vi "IsolateError.vi"(8 "Err Line":i32=71, 9 "Number of lines":i32=71, 10 "start":i32=1390, 11 "Console in":string=">>> \n>>> \nHUB: sync filesystems\nHUB: soft reboot\nTraceback (most recent call last):\n  File \"main.py\", line 81, in <module>\nKeyboardInterrupt: \nMicroPython v1.14-875-g1ed8d92bd on 2021-04-23; LEGO Technic Small Hub with STM32F413xx\nType \"help()\" for more information.\n>>> \nHUB: sync filesystems\nHUB: soft reboot\nTraceback (most recent call last):\n  File \"main.py\", line 81, in <module>\nKeyboardInterrupt: \nMicroPython v1.14-875-g1ed8d92bd on 2021-04-23; LEGO Technic Small Hub with STM32F413xx\nType \"help()\" for more information.\n>>> \n>>> \n>>> \n>>> \n>>> >>> \nHUB: sync filesystems\nHUB: soft reboot\nTraceback (most recent call last):\n  File \"main.py\", line 71, in <module>\n  File \"Backpack_Code.py\", line 81, in ask\n  File \"Backpack_Code.py\", line 56, in upload\n  File \"Backpack_Code.py\", line 25, in read\nKeyboardInterrupt: \nMicroPython v1.14-875-g1ed8d92bd on 2021-04-23; LEGO Technic Small Hub with STM32F413xx\nType \"help()\" for more information.\n>>> \n>>> \n>>> hub.\n__class__       __name__        __version__     BACK\nBOTTOM          BT_VCP          FRONT           LEFT\nRIGHT           TOP             USB_VCP         battery\nbluetooth       button          config          file_transfer\ninfo            led             motion          port\npower_off       repl_restart    reset           status\nsupervision     temperature\n>>> hub.led(2)\n>>> hub.led(4)\n>>> hub.led(6)\n>>> hub.led(8)\n>>> >>> \nHUB: sync filesystems\nHUB: soft reboot\nTraceback (most recent call last):\n  File \"main.py\", line 71\nSyntaxError: invalid syntax\nMicroPython v1.14-875-g1ed8d92bd on 2021-04-23; LEGO Technic Small Hub with STM32F413xx\nType \"help()\" for more information.\n>>> import hub\n>>> import utime\n>>> from Backpack_Code import Backpack\n>>> SSID = 'Tufts_Wireless'\n>>> PSWD = ''\n>>> CAR = 'fl'\n>>> commands = '''\n... \\x05\n... import utime\n... from umqtt.simple import MQTTClient\n... import network,machine,ubinascii\n... LED = machine.Pin(2, machine.Pin.OUT)\n... speed = 0\n... MQTT = {\n... \"MQTT_BROKER\" : \"10.245.82.149\",\n... \"PORT\" : 1883,\n... \"TOPIC\" : 'car/%s',\n... \"CLIENT_ID\" : ubinascii.hexlify(machine.unique_id())\n... \n... }\n... def wifi(SSID,KEY):\n...     wlan = network.WLAN()\n...     wlan.active(True)\n...     wlan.connect(SSID, KEY)\n...     mac = ubinascii.hexlify(network.WLAN().config('mac'),':').decode()\n...     print(\"MAC \" + mac)\n...     while '0.0.0.0' in wlan.ifconfig():\n...         utime.sleep(1)\n...     return wlan.ifconfig()\n... \n... def GotIt(topic, msg):\n...     global speed\n...     if topic.decode('utf-8') == MQTT[\"TOPIC\"]:\n...         oldspeed = speed\n...         speed = int(msg)\n...         if oldspeed != speed:\n...             print(speed)\n... \n... def mqtt():\n...     client = MQTTClient(client_id = MQTT[\"CLIENT_ID\"], server = MQTT[\"MQTT_BROKER\"], port = MQTT[\"PORT\"])\n...     client.set_callback(GotIt)\n...     client.connect()\n...     return client\n... \n... LED.off()\n... ip = wifi('%s','%s')\n... print(ip)\n... LED.on()\n... client = mqtt()\n... client.subscribe(MQTT[\"TOPIC\"])\n... client.publish('car/name',MQTT[\"TOPIC\"])\n... \\x04\n... '''\n>>> commands = commands % (CAR,SSID,PSWD)\n>>> def configure():\n...     if not dongle.setup(): return False\n...     for cmd in commands.split('\\n'):\n...         if not dongle.EOL(dongle.ask(cmd)) : return False\n...     return True\n... \n>>> hub.led(2)\n>>> dongle = Backpack(hub.port.B, verbose = False)\n>>> print(dongle.setup()\n... hub.led(4)\n... if configure():\n...     while True:\n...         hub.led(8)\n...         fred = dongle.ask('client.check_msg()')\n...         fred += dongle.ask()\n...         fred = fred.split('\\r\\n')\n...         hub.led(6)\n...         if len(fred) > 3:\n...             fred = fred[1:-2]\n...             fred = [int(i) for i in fred]\n...             print(fred)\n...             hub.port.A.motor.pwm(fred[-1])\n...         else:\n...             utime.sleep(0.1)\n...             \n...             \n... \n... \n... \n... \n... ") -> (0 "line coord":cluster{"Start":i32, "end":i32}={"Start"=3360, "end"=3385}, 1 "Line length":i32=24, 2 "substring":string=">>> print(dongle.setup()", 3 "EOL":i32=3385, 4 "Line info":T1={"line number"=71, "Error"=">>> print(dongle.setup()", {"Start"=3360, "end"=3385}}, 5 "success?":bool=TRUE)   [LabVIEW 2022 SP3]
panel:
  out "substring 2":string=" >>> \nHUB: sync filesystems\nHUB: soft reboot\nTraceback (most recent call last):\n  File \"main.py\", line 71\nSyntaxError: invalid syntax\nMicroPython v1.14-875-g1ed8d92bd on 2021-04-23; LEGO Technic Small Hub with STM32F413xx\nType \"help()\" for more information.\n>>> import hub\n>>> import utime\n>>> from Backpack_Code import Backpack\n>>> SSID = 'Tufts_Wireless'\n>>> PSWD = ''\n>>> CAR = 'fl'\n>>> commands = '''\n... \\x05\n... import utime\n... from umqtt.simple import MQTTClient\n... import network,machine,ubinascii\n... LED = machine.Pin(2, machine.Pin.OUT)\n... speed = 0\n... MQTT = {\n... \"MQTT_BROKER\" : \"10.245.82.149\",\n... \"PORT\" : 1883,\n... \"TOPIC\" : 'car/%s',\n... \"CLIENT_ID\" : ubinascii.hexlify(machine.unique_id())\n... \n... }\n... def wifi(SSID,KEY):\n...     wlan = network.WLAN()\n...     wlan.active(True)\n...     wlan.connect(SSID, KEY)\n...     mac = ubinascii.hexlify(network.WLAN().config('mac'),':').decode()\n...     print(\"MAC \" + mac)\n...     while '0.0.0.0' in wlan.ifconfig():\n...         utime.sleep(1)\n...     return wlan.ifconfig()\n... \n... def GotIt(topic, msg):\n...     global speed\n...     if topic.decode('utf-8') == MQTT[\"TOPIC\"]:\n...         oldspeed = speed\n...         speed = int(msg)\n...         if oldspeed != speed:\n...             print(speed)\n... \n... def mqtt():\n...     client = MQTTClient(client_id = MQTT[\"CLIENT_ID\"], server = MQTT[\"MQTT_BROKER\"], port = MQTT[\"PORT\"])\n...     client.set_callback(GotIt)\n...     client.connect()\n...     return client\n... \n... LED.off()\n... ip = wifi('%s','%s')\n... print(ip)\n... LED.on()\n... client = mqtt()\n... client.subscribe(MQTT[\"TOPIC\"])\n... client.publish('car/name',MQTT[\"TOPIC\"])\n... \\x04\n... '''\n>>> commands = commands % (CAR,SSID,PSWD)\n>>> def configure():\n...     if not dongle.setup(): return False\n...     for cmd in commands.split('\\n'):\n...         if not dongle.EOL(dongle.ask(cmd)) : return False\n...     return True\n... \n>>> hub.led(2)\n>>> dongle = Backpack(hub.port.B, verbose = False)\n>>> print(dongle.setup()\n... hub.led(4)\n... if configure():\n...     while True:\n...         hub.led(8)\n...         fred = dongle.ask('client.check_msg()')\n...         fred += dongle.ask()\n...         fred = fred.split('\\r\\n')\n...         hub.led(6)\n...         if len(fred) > 3:\n...             fred = fred[1:-2]\n...             fred = [int(i) for i in fred]\n...             print(fred)\n...             hub.port.A.motor.pwm(fred[-1])\n...         else:\n...             utime.sleep(0.1)\n...             \n...             \n... \n... \n... \n... \n... "
  out "Array":string[](array[string])=[" >>> \n", "HUB: sync filesystems\n", "HUB: soft reboot\n", "Traceback (most recent call last):\n", "  File \"main.py\", line 71\n", "SyntaxError: invalid syntax\n", "MicroPython v1.14-875-g1ed8d92bd on 2021-04-23; LEGO Technic Small Hub with STM32F413xx\n", "Type \"help()\" for more information.\n", ">>> import hub\n", ">>> import utime\n", ">>> from Backpack_Code import Backpack\n", ">>> SSID = 'Tufts_Wireless'\n", ">>> PSWD = ''\n", ">>> CAR = 'fl'\n", ">>> commands = '''\n", "... \\x05\n", "... import utime\n", "... from umqtt.simple import MQTTClient\n", "... import network,machine,ubinascii\n", "... LED = machine.Pin(2, machine.Pin.OUT)\n", "... speed = 0\n", "... MQTT = {\n", "... \"MQTT_BROKER\" : \"10.245.82.149\",\n", "... \"PORT\" : 1883,\n", "... \"TOPIC\" : 'car/%s',\n", "... \"CLIENT_ID\" : ubinascii.hexlify(machine.unique_id())\n", "... \n", "... }\n", "... def wifi(SSID,KEY):\n", "...     wlan = network.WLAN()\n", "...     wlan.active(True)\n", "...     wlan.connect(SSID, KEY)\n", "...     mac = ubinascii.hexlify(network.WLAN().config('mac'),':').decode()\n", "...     print(\"MAC \" + mac)\n", "...     while '0.0.0.0' in wlan.ifconfig():\n", "...         utime.sleep(1)\n", "...     return wlan.ifconfig()\n", "... \n", "... def GotIt(topic, msg):\n", "...     global speed\n", "...     if topic.decode('utf-8') == MQTT[\"TOPIC\"]:\n", "...         oldspeed = speed\n", "...         speed = int(msg)\n", "...         if oldspeed != speed:\n", "...             print(speed)\n", "... \n", "... def mqtt():\n", "...     client = MQTTClient(client_id = MQTT[\"CLIENT_ID\"], server = MQTT[\"MQTT_BROKER\"], port = MQTT[\"PORT\"])\n", "...     client.set_callback(GotIt)\n", "...     client.connect()\n", "...     return client\n", "... \n", "... LED.off()\n", "... ip = wifi('%s','%s')\n", "... print(ip)\n", "... LED.on()\n", "... client = mqtt()\n", "... client.subscribe(MQTT[\"TOPIC\"])\n", "... client.publish('car/name',MQTT[\"TOPIC\"])\n", "... \\x04\n", "... '''\n", ">>> commands = commands % (CAR,SSID,PSWD)\n", ">>> def configure():\n", "...     if not dongle.setup(): return False\n", "...     for cmd in commands.split('\\n'):\n", "...         if not dongle.EOL(dongle.ask(cmd)) : return False\n", "...     return True\n", "... \n", ">>> hub.led(2)\n", ">>> dongle = Backpack(hub.port.B, verbose = False)\n", ">>> print(dongle.setup()\n"]
  out "Waveform Graph":i32[](graph)=[6, 22, 17, 35, 26, 28, 88, 36, 15, 17, 39, 28, 14, 15, 19, 9, 17, 40, 37, 42, 14, 13, 37, 19, 24, 57, 5, 6, 24, 30, 26, 32, 75, 28, 44, 27, 31, 5, 27, 21, 51, 29, 29, 34, 29, 5, 16, 110, 35, 25, 22, 5, 14, 25, 14, 13, 20, 36, 45, 9, 8, 42, 21, 44, 41, 62, 20, 5, 15, 51, 25]
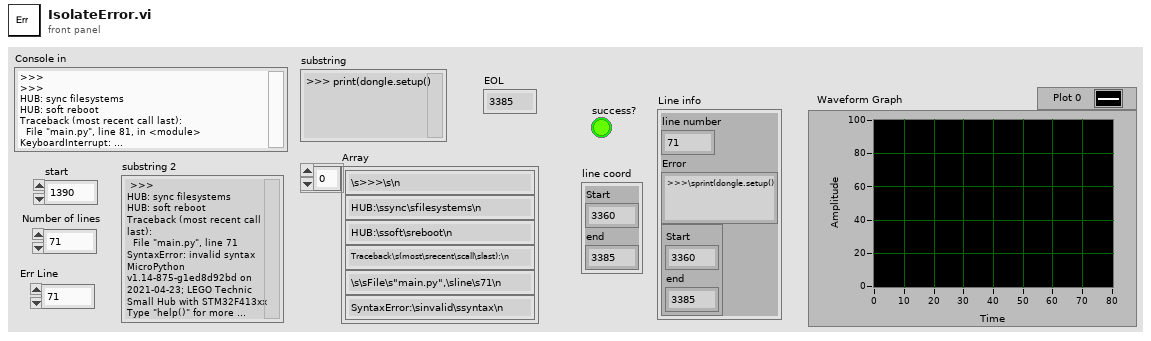
[diagram p1: front panel]
types:
  T1 = cluster{"line number":i32, "Error":string, cluster{"Start":i32, "end":i32}}
  T2 = cluster{"Number of lines":i32, "Console in":string, cluster{"start":i32, "offset past match":i32}}
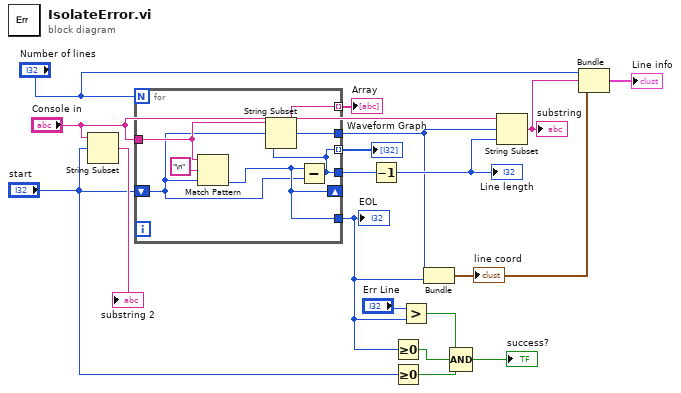
[diagram p0: block diagram]
diagram:
  n1 = String Subset(string="Console in", offset (0)="start") -> (substring=→"substring 2":string)  [unwired: 1 in]
  n2 = for {
    N: "Number of lines" -> [_]
    tunnel: "Console in" -> [w22]
    shift-right: [w23] -> _
    shift-left: "start" -> [w19]
    tunnel: [w21] -> w16
    tunnel: [w23] -> w1
    tunnel: [w21] -> w10 mode=indexing
    tunnel: [w20] -> w9 mode=indexing
    tunnel: [w19] -> w8
    n3 = Match Pattern(string=w22, regular expression="\n", offset (0)=w19) -> (offset past match=w23:i32)  [unwired: 3 out]
    n4 = Subtract(x=w23, y=w19) -> (x-y=w21:i32)
    n5 = String Subset(string=w22, offset (0)=w19, length (rest)=w21) -> (substring=w20:string)
  }
  "EOL" <- w1
  "Waveform Graph" <- w10
  "Array" <- w9
  n6 = Decrement(x=w16) -> (x-1=w11:i32)
  "Line length" <- w11
  n7 = Greater Or Equal To 0?(x=w1) -> (x >= 0?=w18:bool)
  n8 = Greater Or Equal To 0?(x="start") -> (x >= 0?=w17:bool)
  n9 = Greater?(x="Err Line", y=w1) -> (0:w3:bool)
  n10 = Bundle("start"=w8, "offset past match"=w1) -> (w14:cluster{"start":i32, "offset past match":i32})  [unwired: 1 in]
  "line coord" <- w14
  n11 = Compound Arithmetic op=AND(w3, w18, w17) -> (→"success?":bool)
  n12 = String Subset(string="Console in", offset (0)=w8, length (rest)=w11) -> (substring=w15:string)
  "substring" <- w15
  n13 = Bundle("Number of lines"="Number of lines", "Console in"=w15, w14) -> (→"Line info":T2)  [unwired: 1 in]
